vi "Write to HDF File.vi"(7 "indices":i32[](array[numeric]), 8 "error in (no error)":errorcluster, 10 "My Type":T1, 11 "path":path) -> (0 "error out":errorcluster)   [LabVIEW 2019, in "HDF5 Tools.lvlib"]
uses:
  mytype.ctl
  <vilib>/UPVI/lvhdf5/file.llb/LVH5F Operation.ctl
  HDF5 Tools.lvlib
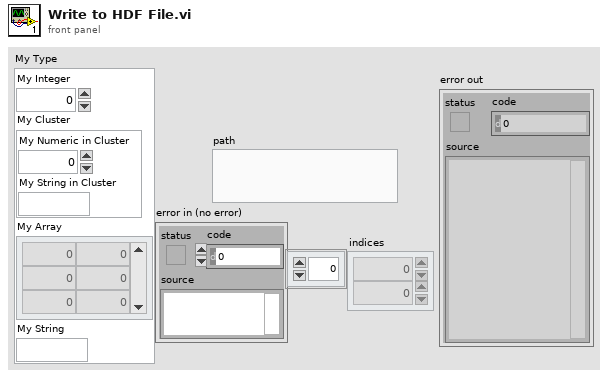
[diagram p1: front panel]
types:
  T1 = typedef "mytype.ctl" = cluster{"My Integer":i32, "My Cluster":cluster{"My Numeric in Cluster":dbl, "My String in Cluster":string}, "My Array":i32[][], "My String":string}
  T2 = typedef "LVH5F Operation.ctl" = enum16{"open", "open or create", "create or replace", "create or replace (with confirmation)", "create", "open (read only)"}
  T3 = typedef "HDF5 Ref.ctl" = refnum<k1>
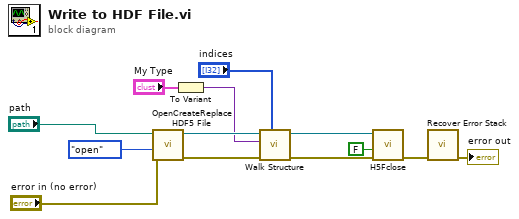
[diagram p0: block diagram]
diagram:
  n1 = call <vilib>:"OpenCreateReplace HDF5 File.vi"("error in (no error)"="error in (no error)", "function (open or create)"=LVH5F_Operation."open", "path"="path") -> ("error out"=w9:errorcluster, "HDF5 Ref out"=w11:T3)  [unwired: 5 in]
  n2 = To Variant(anything="My Type") -> (Variant=w6:variant)
  n3 = call "Walk Structure.vi"("indices"="indices", "error in (no error)"=w9, "variant"=w6, "Refnum in"=w11) -> ("error out"=w8:errorcluster, "Refnum out"=w10:T3)  [unwired: 4 in]
  n4 = call <vilib>:"H5Fclose.vi"("error in (no error)"=w8, "Force Close (F)"=FALSE, "HDF5 Ref"=w10) -> ("error out"=w13:errorcluster)  [unwired: 6 in]
  n5 = call <vilib>:"Recover Error Stack.vi"("error in (no error)"=w13) -> ("error out"=→"error out":errorcluster)  [unwired: 5 in, 3 out]
